vi "ReservWL.vi"(1 "Tags":i32[](array[numeric]), 2 "ArrayIn":waveform(i16)[](array[waveform]), 3 "t1-t0":dbl) -> (0 "Array":waveform(i16)[](array[waveform]))   [LabVIEW 2010]
uses:
  70user.lib/TheSigTab.vi
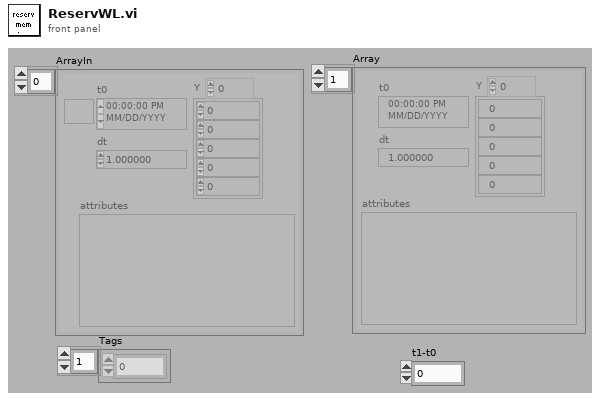
[diagram p1: front panel]
types:
  T1 = cluster{"s_Type":u16, "FIFO":u16, "IrqStep":u16, "Pages":u16, "AutoInit":u16, "dRate":dbl, "dKadr":dbl, "dScale":dbl, "Rate":u16, "Kadr":u16, "Scale":u16, "FPDelay":u16, "SynchroType":u16, "SynchroSensitivity":u16, "SynchroMode":u16, "AdChannel":u16, "AdPorog":u16, "NCh":u16, "Chn":i32[], "IrqEna":u16, "AdcEna":u16}
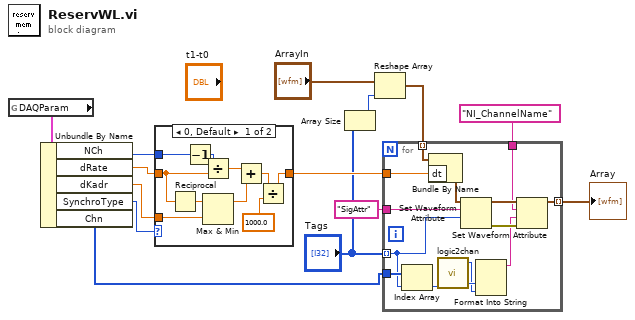
[diagram p0: block diagram]
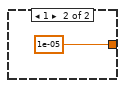
[diagram p2: hidden frame]
diagram:
  n1 = global read "TheSigTab.vi" "DAQParam"() -> (w10:T1)
  n2 = Unbundle By Name(w10) -> ("NCh"=w8:u16, "dRate"=w12:dbl, "dKadr"=w13:dbl, "SynchroType"=w11:u16, "Chn"=w6:i32[])
  n3 = case shown="0, Default" w11 {
    tunnel: w13 -> [w20 _]
    tunnel: w12 -> [w21 _]
    tunnel: w8 -> [w24 _]
    tunnel: [w16 1e-05] -> w2
    frame 0, Default {
      n4 = Reciprocal(x=w21) -> (1/x=w18:dbl)
      n5 = Decrement(x=w24) -> (x-1=w23:u16)
      n6 = Divide(x=w23, y=w21) -> (x/y=w22:dbl)
      n7 = Max & Min(x=w18, y=w20) -> (max(x,y)=w19:dbl)  [unwired: 1 out]
      n8 = Add(x=w22, y=w19) -> (x+y=w17:dbl)
      n9 = Divide(x=w17, y=1000.0) -> (x/y=w16:dbl)
    }
    frame 1 {
    }
  }
  n10 = Array Size(array="Tags") -> (size(s)=w3:i32)
  n11 = Reshape Array("ArrayIn", w3) -> (w4:waveform(i16)[])
  n12 = for {
    tunnel: [w34] -> w14 mode=indexing
    tunnel: w2 -> [w39]
    tunnel: "SigAttr" ("name") -> [w37]
    tunnel: "NI_ChannelName" -> [w33]
    tunnel: w6 -> [w29]
    tunnel: "Tags" -> [w27] mode=indexing
    tunnel: w4 -> [w26] mode=indexing
    n13 = Index Array(array=w29, index=w27) -> (element=w28:i32)
    n14 = Bundle By Name(cluster=w26, "dt"=w39) -> (w38:waveform(i16))
    n15 = call "logic2chan.vi"("value"=w28) -> ("Канал"=w31:u8, "Switch"=w32:enum16{"X-Y", "На землю", "X", "Y"})  [unwired: 1 out]
    n16 = Set Waveform Attribute(5:w27, 6:w37, 7:w38) -> (0:w36:errorcluster, 3:w35:waveform(i16))  [unwired: 1 in, 1 out]
    n17 = Format Into String(w32, w31) -> (resulting string=w30:string)  [unwired: 3 in, 1 out]
    n18 = Set Waveform Attribute(4:w36, 5:w30, 6:w33, 7:w35) -> (3:w34:waveform(i16))  [unwired: 2 out]
  }
  "Array" <- w14
